vi "Disconnect.vi"(8 "Error In":errorcluster, 10 "Description":string="Normal Shutdown", 11 "Session In":refnum<class "Session.lvclass">) -> (0 "Error Out":errorcluster, 3 "Sesssion Out":refnum<class "Session.lvclass">)   [LabVIEW 2017, in "LabSSH2.lvlib" / "Session.lvclass"]
uses:
  Session.lvclass
  Session.lvclass/Session.ctl
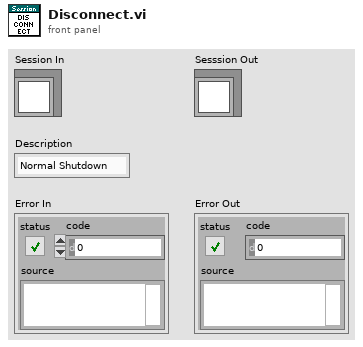
[diagram p1: front panel]
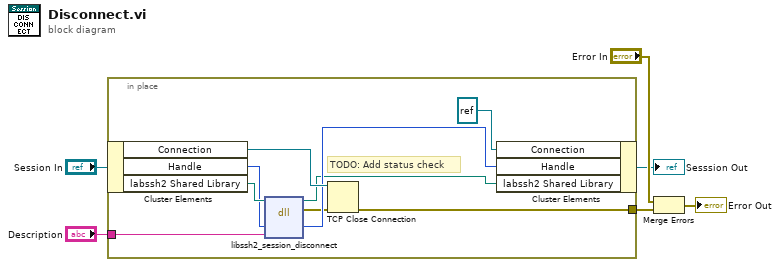
[diagram p0: block diagram]
diagram:
  n1 = in-place {
    in-place-border: "Description" -> [w13]
    in-place-border: [w10] -> w1
    # "TODO: Add status check"
    n2 = in-place-cluster #1("Session In") -> ("Connection"=w15:refnum<k5>, "Handle"=w7:u64, "labssh2 Shared Library"=w8:path)
    n3 = dll-call lib="D:/Users/cfield/Code/Field R&D Services/SSH/LabSSH2/LabVIEW/trunk/src/LabSSH2/Private/labssh2.*" fn="libssh2_session_disconnect"(path in=w8, "session"=w7, "description"=w13) -> (path out=w11:path, error out=w9:errorcluster, "session"=w12:u64)  [unwired: 4 in]
    n4 = TCP Close Connection(connection ID=w15, error in (no error)=w9) -> (error out=w10:errorcluster)  [unwired: 1 in, 1 out]
    n5 = in-place-cluster #1("Connection"=refnum<k5> refnum, "Handle"=w12, "labssh2 Shared Library"=w11) -> (→"Sesssion Out":refnum<class "Session.lvclass">)
  }
  n6 = Merge Errors("Error In", w1) -> (→"Error Out":errorcluster)
